vi "Perform Decimation Test.vi"(4 "Expected Group dts":dbl[](array[numeric]), 6 "Expected Y Array Sizes":i32[](array[numeric]), 7 "Decimation":dbl, 8 "error in":errorcluster, 9 "Embedded Data Logger Channel Group Name":string, 10 "Embedded Data Logger File Name":string, 11 "Embedded Data Logger Windows System Tests in":refnum<class "Embedded Data Logger Windows System Tests.lvclass">) -> (0 "error out":errorcluster, 3 "Embedded Data Logger Windows System Tests out":refnum<class "Embedded Data Logger Windows System Tests.lvclass">)   [LabVIEW 2019, in "Embedded Data Logger Windows System Tests.lvclass"]
uses:
  Embedded Data Logger Windows System Tests.lvclass
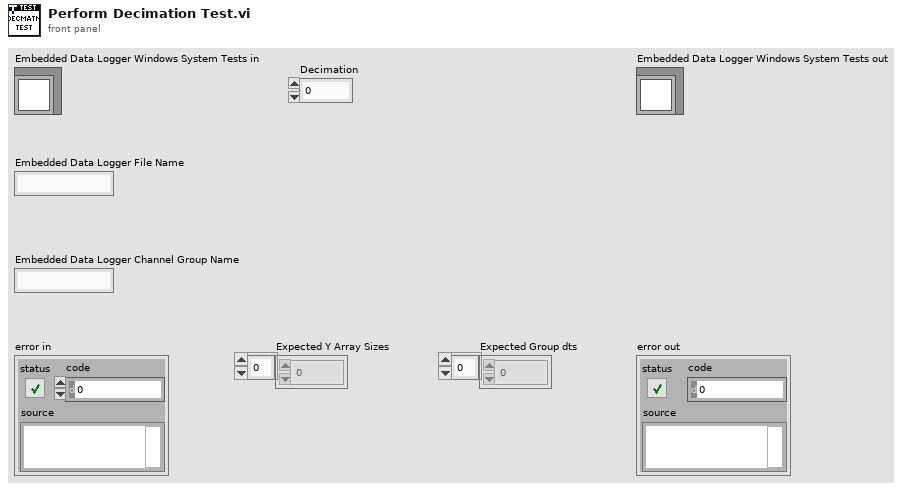
[diagram p1: front panel]
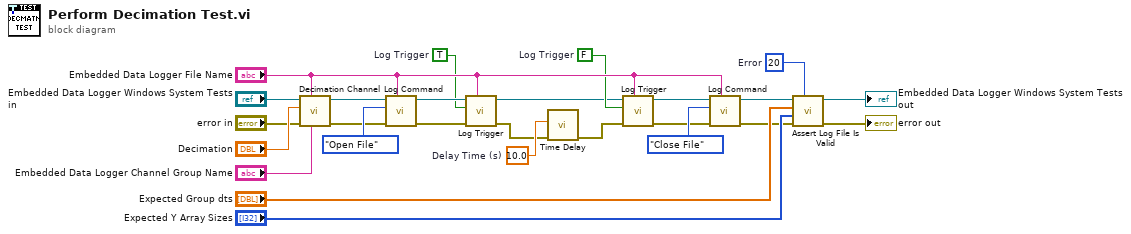
[diagram p0: block diagram]
diagram:
  w12 = 20  # Error
  w8 = FALSE  # Log Trigger
  w7 = 10.0  # Delay Time (s)
  w5 = TRUE  # Log Trigger
  n1 = call "Decimation Channel.vi"("Embedded Data Logger Channel Group Name"="Embedded Data Logger Channel Group Name", "Embedded Data Logger File Name"="Embedded Data Logger File Name", "error in"="error in", "Decimation"="Decimation", "Embedded Data Logger System Tests in"="Embedded Data Logger Windows System Tests in") -> ("error out"=w19:errorcluster, "Embedded Data Logger System Tests out"=w21:refnum<class "Embedded Data Logger Windows System Tests.lvclass">)  [unwired: 5 in]
  n2 = call "Log Command.vi"("Embedded Data Logger File Name"="Embedded Data Logger File Name", "error in"=w19, "Log Command"=enum16{"Idle", "Open File", "Close File"}."Open File", "Embedded Data Logger System Tests in"=w21) -> ("error out"=w20:errorcluster, "Embedded Data Logger System Tests out"=w22:refnum<class "Embedded Data Logger Windows System Tests.lvclass">)  [unwired: 6 in]
  n3 = call "Log Trigger.vi"("Embedded Data Logger File Name"="Embedded Data Logger File Name", "error in"=w20, "Log Trigger"=w5, "Embedded Data Logger System Tests in"=w22) -> ("error out"=w4:errorcluster, "Embedded Data Logger System Tests out"=w3:refnum<class "Embedded Data Logger Windows System Tests.lvclass">)  [unwired: 6 in]
  n4 = call "Time Delay"("error in (no error)"=w4, "Delay Time (s)"=w7) -> ("error out"=w6:errorcluster)  [unwired: 9 in]
  n5 = call "Log Trigger.vi"("Embedded Data Logger File Name"="Embedded Data Logger File Name", "error in"=w6, "Log Trigger"=w8, "Embedded Data Logger System Tests in"=w3) -> ("error out"=w1:errorcluster, "Embedded Data Logger System Tests out"=w2:refnum<class "Embedded Data Logger Windows System Tests.lvclass">)  [unwired: 6 in]
  n6 = call "Log Command.vi"("Embedded Data Logger File Name"="Embedded Data Logger File Name", "error in"=w1, "Log Command"=enum16{"Idle", "Open File", "Close File"}."Close File", "Embedded Data Logger System Tests in"=w2) -> ("error out"=w11:errorcluster, "Embedded Data Logger System Tests out"=w9:refnum<class "Embedded Data Logger Windows System Tests.lvclass">)  [unwired: 6 in]
  n7 = call "Assert Log File Is Valid.vi"("Error"=w12, "error in"=w11, "Expected Y Array Sizes"="Expected Y Array Sizes", "Expected Group dts"="Expected Group dts", "Embedded Data Logger System Tests in"=w9) -> ("error out"=→"error out":errorcluster, "Embedded Data Logger System Tests out"=→"Embedded Data Logger Windows System Tests out":refnum<class "Embedded Data Logger Windows System Tests.lvclass">)  [unwired: 5 in]
